vi "List Platform Applications.vi"(8 "error in (no error)":errorcluster, 10 "Region":T1, 11 "AWS Credentials":T2) -> (0 "error out":errorcluster, 3 "Platform Applications out":refnum<class "Platform Application.lvclass">[](array[class]))   [LabVIEW 2015, in "NI_AWS_SNS.lvlib" / "Platform Application.lvclass"]
doc: "Lists the platform application objects for the supported push notification services, such as APNS and GCM."
uses:
  Platform Application.lvclass
  Core/HTTP Request/AWS Credentials.ctl
  Core/HTTP Request/Region.ctl
  Core/HTTP Request/HTTP Request.lvclass/HTTP Request.ctl
  Core/HTTP Request/Write Credentials.vi
  Core/HTTP Request/Write Region.vi
  Core/HTTP Request/Write Service.vi
  Core/HTTP Request/Write Verify Server.vi
  Core/ARN/ARN.lvclass
  Core/HTTP Request/HTTP Request.lvclass
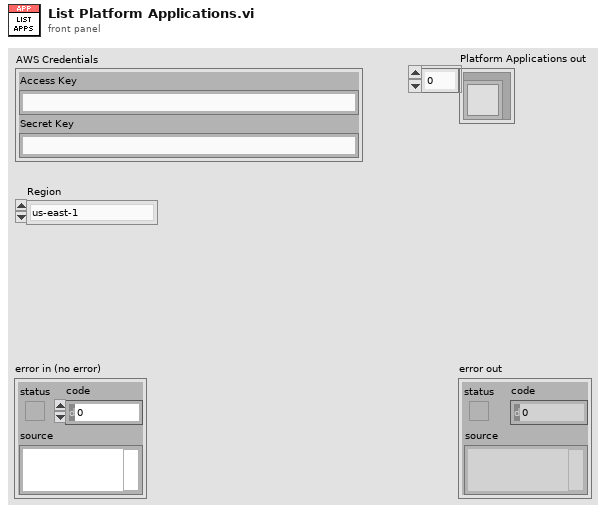
[diagram p1: front panel]
types:
  T1 = typedef "NI_AWS_Core.lvlib/HTTP Request.lvclass/Region.ctl" = enum16{"us-east-1", "us-east-2", "us-west-1", "us-west-2", "ap-northeast-1", "ap-northeast-2", "ap-southeast-1", "ap-southeast-2", "ca-central-1", "eu-central-1", "eu-west-1", "eu-west-2", "sa-east-1"}
  T2 = typedef "NI_AWS_Core.lvlib/HTTP Request.lvclass/AWS Credentials.ctl" = cluster{"Access Key":string, "Secret Key":string}
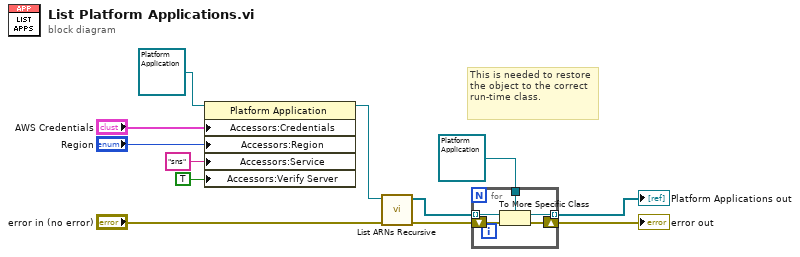
[diagram p0: block diagram]
diagram:
  # "This is needed to restore the object to the correct run-time class."
  n1 = property class="Platform Application"(reference=refnum<class "Platform Application.lvclass"> refnum ("NI_AWS_SNS.lvlib:Platform Application"), "Accessors:Credentials"="AWS Credentials", "Accessors:Region"="Region", "Accessors:Service"="sns" ("Service"), "Accessors:Verify Server"=TRUE ("Verify Server")) -> (reference out=w10:refnum<class "Platform Application.lvclass">)  [unwired: 1 in, 1 out]
  n2 = call "List ARNs Recursive.vi"("error in (no error)"="error in (no error)", "ARN in"=w10) -> ("error out"=w6:errorcluster, "ARNs out"=w8:refnum<class "ARN.lvclass">[])  [unwired: 8 in]
  n3 = for {
    tunnel: refnum<class "Platform Application.lvclass"> refnum ("NI_AWS_SNS.lvlib:Platform Application") -> [w17]
    tunnel: w8 -> [w16] mode=indexing
    tunnel: [w15] -> w1 mode=indexing
    shift-right: [w13] -> w2
    shift-left: w6 -> [w14]
    n4 = To More Specific Class(target class=w17, reference=w16, error in=w14) -> (specific class reference=w15:refnum<class "Platform Application.lvclass">, error out=w13:errorcluster)
  }
  "error out" <- w2
  "Platform Applications out" <- w1
